vi "FGV_Button_Press.vi"(5 "Boolean array":bool[](array[boolean]), 7 "Action":enum16{"Read", "Write Stop", "Write Result"}(ring), 9 "Boolean In":bool, 11 "Error In":errorcluster) -> (6 "Boolean Array Out":bool[](array[boolean]), 10 "Boolean Out":bool, 15 "Error Out":errorcluster)   [LabVIEW 2016]
doc: "This VI gets or sets the stop user event reference."
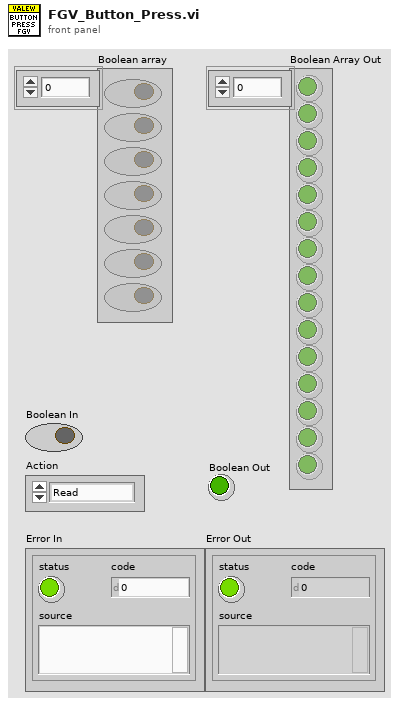
[diagram p1: front panel]
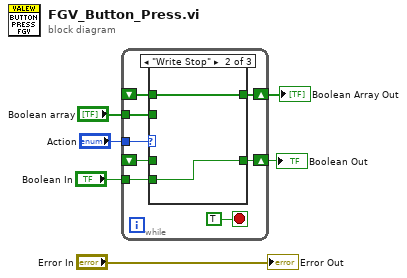
[diagram p0: block diagram]
diagram:
  n1 = while {
    tunnel: "Action" -> [w13]
    tunnel: "Boolean In" -> [w12]
    shift-right: [w11] -> w4
    shift-left: _ -> [w10]
    shift-right: [w9] -> w1
    shift-left: _ -> [w8]
    tunnel: "Boolean array" -> [w7]
    stop <- TRUE stop-if-true
    n2 = case shown="\"Write Stop\"" w13 {
      tunnel: w12 -> [_ w18 _]
      tunnel: [w16 w18 w19] -> w11
      tunnel: w10 -> [w16 _ w19]
      tunnel: [w15 w17 w20] -> w9
      tunnel: w8 -> [w15 w17 _]
      tunnel: w7 -> [_ _ w20]
      frame "Read" {
      }
      frame "Write Stop" {
      }
      frame "Write Result" {
      }
    }
  }
  "Boolean Out" <- w4
  "Boolean Array Out" <- w1
  "Error Out" <- "Error In"
